vi "Compute.vi"(8 "error in (no error)":errorcluster, 9 "Data Channels":T1, 10 "x-var":dbl, 11 "Plus in":refnum<class "Plus.lvclass">) -> (0 "error out":errorcluster, 1 "Add'l Data Channels":T1, 3 "Plus out":refnum<class "Plus.lvclass">)   [LabVIEW 2009, in "Plus.lvclass"]
doc: "Given a data channel and an x-coordinate, compute and return one or more new data channels."
uses:
  Plus.lvclass
  Instruments/Utility Classes/Readable/Data Channels.ctl
  Instruments/Utility Classes/Readable/Data Channel.ctl
  Instruments/Utility Classes/Readable/Data Point.ctl
  Instruments/Utility Classes/Readable/Readable.lvclass
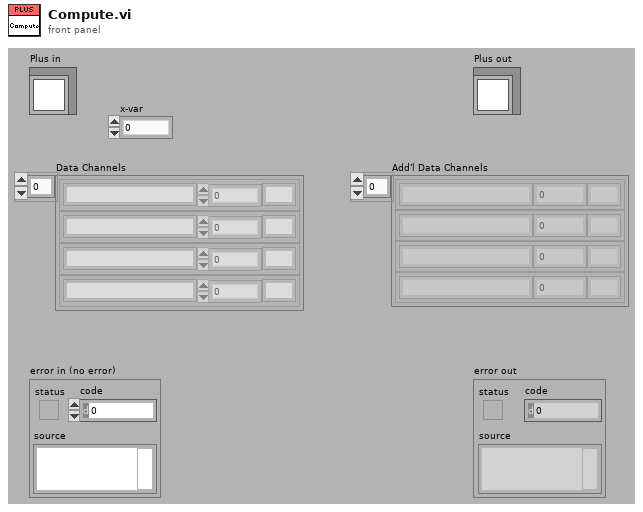
[diagram p1: front panel]
types:
  T1 = typedef "Readable.lvclass/Data Channels.ctl" = T2[]
  T2 = typedef "Readable.lvclass/Data Channel.ctl" = cluster{"Name":string, "Data Point":T3, "Unit":string}
  T3 = typedef "Readable.lvclass/Data Point.ctl" = dbl
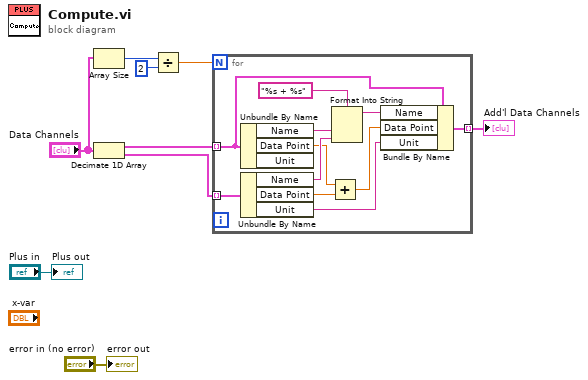
[diagram p0: block diagram]
diagram:
  n1 = Array Size(array="Data Channels") -> (size(s)=w9:i32)
  n2 = Decimate 1D Array "Decimate 1D Array"("Data Channels") -> (w5:T1, w4:T1)
  n3 = Divide(x=w9, y=2) -> (x/y=w8:dbl)
  n4 = for {
    N: w8 -> [_]
    tunnel: w5 -> [w16] mode=indexing
    tunnel: w4 -> [w20] mode=indexing
    tunnel: [w10] -> w1 mode=indexing
    n5 = Unbundle By Name(w16) -> ("Name"=w18:string, "Data Point"=w13:T3)  [unwired: 1 out]
    n6 = Unbundle By Name(w20) -> ("Name"=w17:string, "Data Point"=w12:T3, "Unit"=w15:string)
    n7 = Add(x=w13, y=w12) -> (x+y=w11:T3)
    n8 = Format Into String(format string="%s + %s", w18, w17) -> (resulting string=w14:string)  [unwired: 2 in, 1 out]
    n9 = Bundle By Name(cluster=w16, "Name"=w14, "Data Point"=w11, "Unit"=w15) -> (w10:T2)
  }
  "Add'l Data Channels" <- w1
  "error out" <- "error in (no error)"
  "Plus out" <- "Plus in"
